vi "Log Message.vi"(10 "Message":string, 11 "Log":enum16{"Error Log", "Timer Log", "Scoring Log"}(ring)) -> ()   [LabVIEW 2013]
uses:
  Logfile Entry.ctl
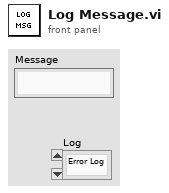
[diagram p1: front panel]
types:
  T1 = typedef "Logfile Entry.ctl" = cluster{"Time Stamp":timestamp, "Origin":string, "Message":string, "Log":enum16{"Error Log", "Timer Log", "Scoring Log"}}
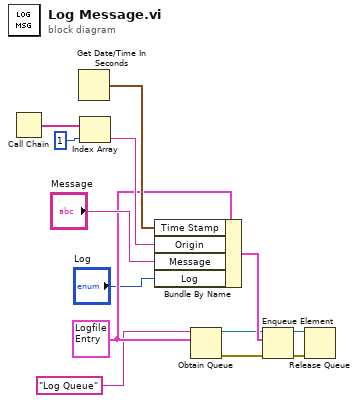
[diagram p0: block diagram]
diagram:
  w7 = T1 {"Time Stamp"=timestamp(0 s since 1904-01-01), "Origin"="", "Message"="", "Log"=enum."Error Log"} ("Cluster")
  n1 = Call Chain() -> (call chain=w11:string[])
  n2 = Get Date/Time In Seconds() -> (seconds since 1Jan1904=w12:timestamp)
  n3 = Index Array(array=w11, index=1) -> (element=w9:string)
  n4 = Bundle By Name(cluster=w7, "Time Stamp"=w12, "Origin"=w9, "Message"="Message", "Log"="Log") -> (w13:T1)
  n5 = Obtain Queue(name (unnamed)="Log Queue", element data type=w7) -> (queue out=w6:refnum<queue>, error out=w5:errorcluster)  [unwired: 3 in, 1 out]
  n6 = Enqueue Element(queue=w6, element=w13, error in (no error)=w5) -> (queue out=w4:refnum<queue>, error out=w3:errorcluster)  [unwired: 1 in, 1 out]
  n7 = Release Queue(queue=w4, error in (no error)=w3) -> ()  [unwired: 1 in, 3 out]
